vi "isExcluded.vi"(8 "error in (no error)":errorcluster, 11 "Goal in":refnum<class "Goal.lvclass">) -> (0 "error out":errorcluster, 2 "Excluded?":bool, 3 "Goal out":refnum<class "Goal.lvclass">)   [LabVIEW 2018, in "Goal.lvclass"]
uses:
  Goal.lvclass
  Goal.lvclass/Goal.ctl
  Category/Category.lvclass
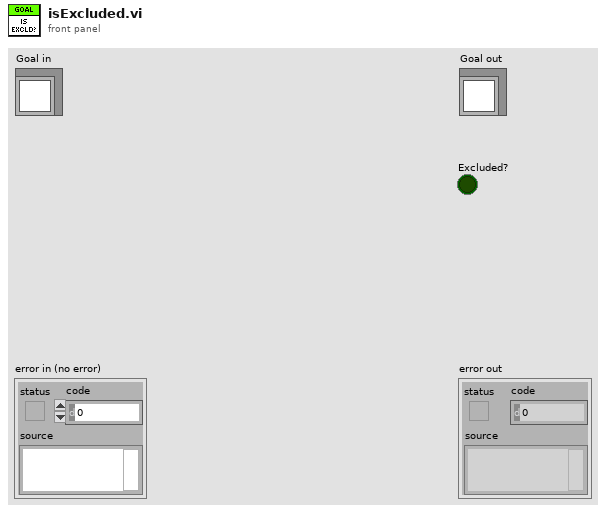
[diagram p1: front panel]
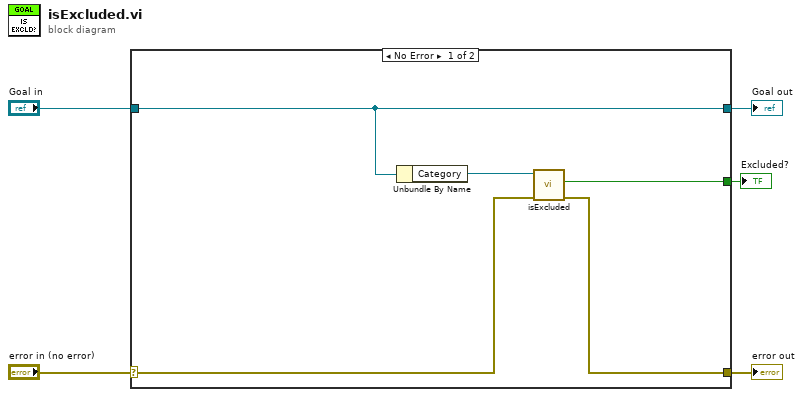
[diagram p0: block diagram]
diagram:
  n1 = case shown="No Error" "error in (no error)" {
    selector: "error in (no error)" -> [w7 w12]
    tunnel: [w6 w12] -> w4
    tunnel: [w10 w11] -> w2
    tunnel: "Goal in" -> [w10 w11]
    tunnel: [w8 _] -> w1
    frame No Error {
      n2 = Unbundle By Name(w10) -> ("Category"=w9:refnum<class "Category.lvclass">)
      n3 = call "isExcluded.vi"("error in (no error)"=w7, "Category in"=w9) -> ("error out"=w6:errorcluster, "Excluded?"=w8:bool)  [unwired: 7 in, 1 out]
    }
    frame Error {
    }
  }
  "error out" <- w4
  "Goal out" <- w2
  "Excluded?" <- w1
